vi "Zaber A Series Streaming.vi"() -> ()   [LabVIEW 2015]
doc: "Streaming lets you queue a number of commands to be completed in series. With multi-axis controllers the movement is co-ordinated to make lines, arcs, or circles. \n\nThis example allows interactive execution of some of the streaming commands. Some of the features will function with single axis streams."
uses:
  Zaber A Series.lvlib
  <vilib>/Utility/file.llb/Read Delimited Spreadsheet (string).vi
  Public/Action-Status/Streaming/Stream Line (FW7).vi
  Public/Action-Status/Streaming/Stream Arc (FW7).vi
  Public/Action-Status/Streaming/Stream Circle (FW7).vi
panel:
  in  "Quit":bool
  in  "End Stream":bool
  in  "Start Stream":bool
  in  "Stop":bool
  in  "Device Number":string
  in  "VISA resource name":refnum<visa-resource-name>
  in  "Home Axes":bool
  out "Port Open":bool
  out "Device supports streams":bool
  in  "Connect":bool
  in  "Close Port":bool
  out "Number of Stream Buffers Available":i32
  out "Number of Streams Available":i32
  in  "Stream Number":u8=1
  in  "Axis Numbers":u8[](array[numeric])=[1, 2]
  in  "Tab Control":enum32{"Stream Commands", "Command List"}(tab)
  in  "Position Units (0: microsteps)":u16(ring) items=["microsteps", "microns", "millimeters", "inches", "degrees"]
  in  "Microstep Size (0)":dbl
  in  "Line Endpoint":i64[](array[numeric])
  in  "Position Mode":u16(ring) items=["Absolute", "Relative"]
  in  "Line":bool
  in  "Circle":bool
  in  "Arc":bool
  in  "Direction":u16(ring) items=["Clockwise", "Counter-Clockwise"]
  in  "Center":i64[](array[numeric])
  in  "Arc End Point":i64[](array[numeric])
  in  "Send Stream List":bool
  in  "Import CSV":bool
  in  "Stream Commands":string[][](table)=[["stream 1 line rel 20000 20000"], ["stream 1 circle rel cw 10000 0"], ["stream 1 wait 2000"], ["stream 1 line abs 0 0"]]
  in  "file path (dialog if empty)":path
  # "(c) 2017 Zaber Technologies.  ALL RIGHTS RESERVED."
  # "This example demonstrates use of live streaming commands. \n\nFirst Open the port and Home all Axes. The VI will confirm if streams are supported on the device.\n\nNext, enter the Device Number, Stream Number (typically 1), and Axis Numbers (if only 1 axis, then right click on the second axis and select 'delete'). Press Start Stream to begin sending movements.\n\nThe Stream Commands tab allows you to send Lines, Arcs, and Circles. The Command List tab allows you to enter a series of stream commands, or load a list of them from a CSV, and run them in sequence."
  # "Movement"
  # "Lines"
  # "Arcs and Circles"
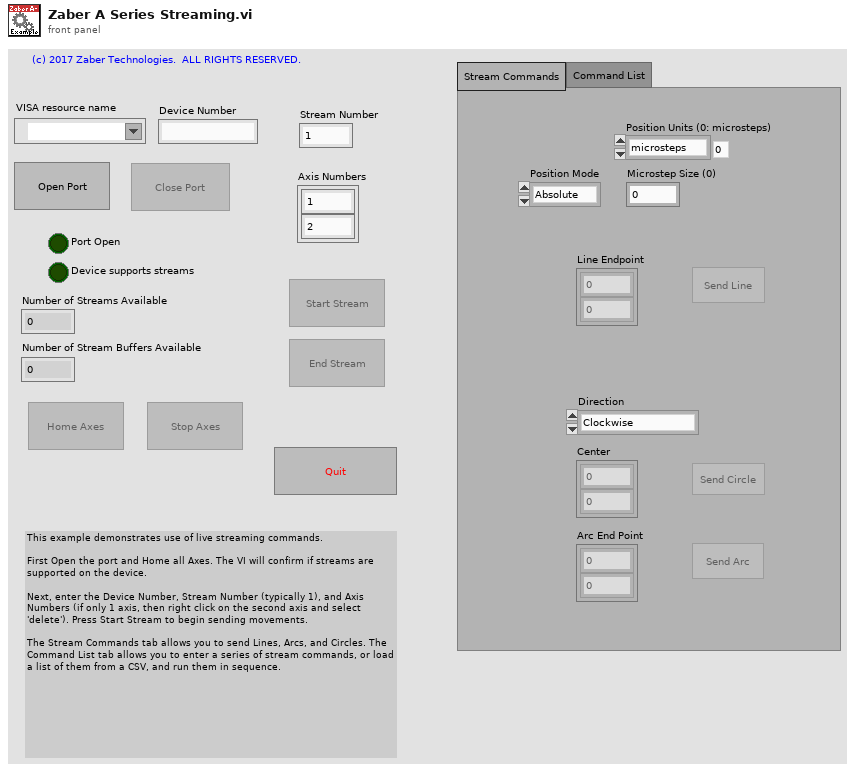
[diagram p1: front panel]
types:
  T1 = enum8{"Enabled", "Disabled", "Disabled and Grayed Out"}
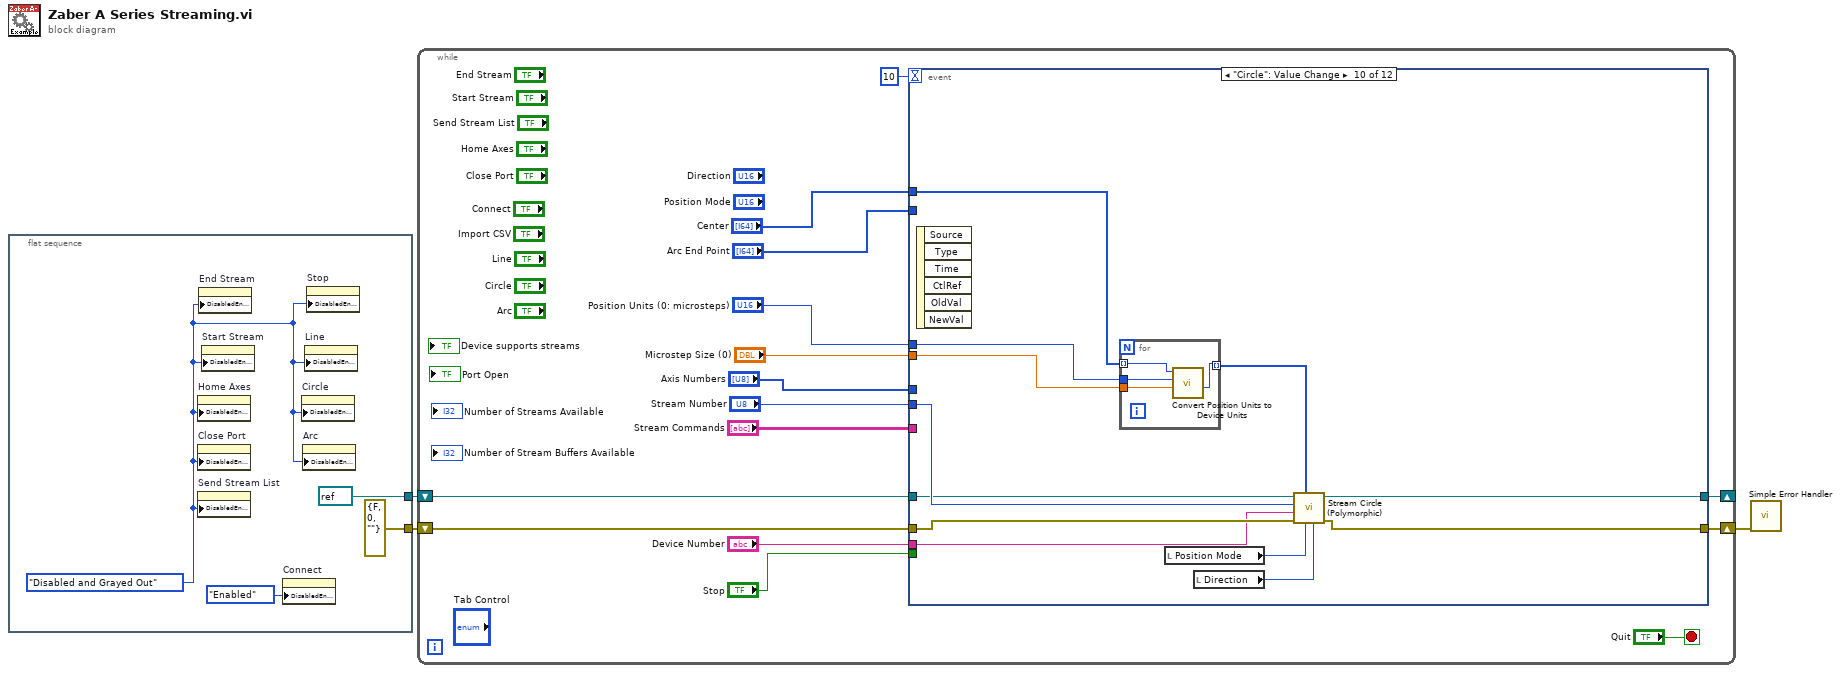
[diagram p0: block diagram]
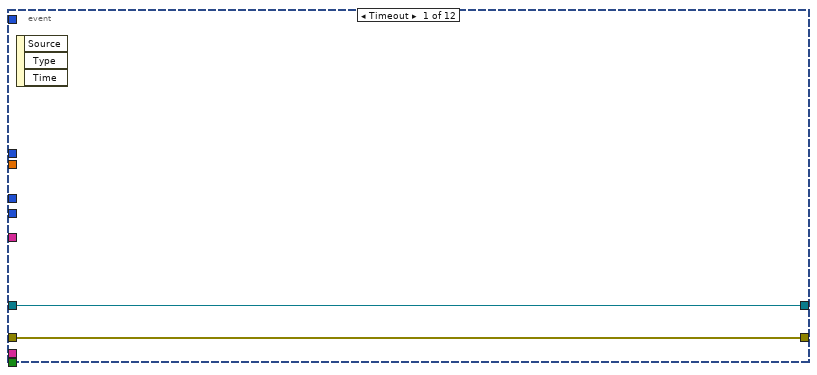
[diagram p2: hidden frame]
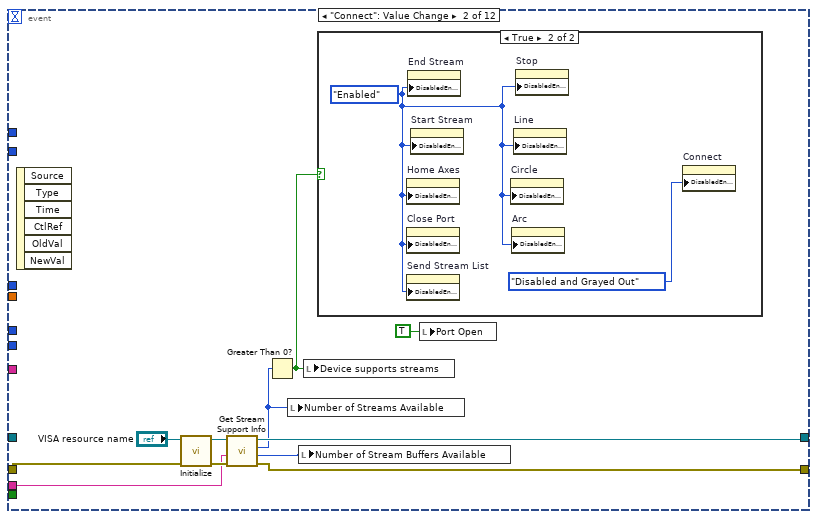
[diagram p3: hidden frame]
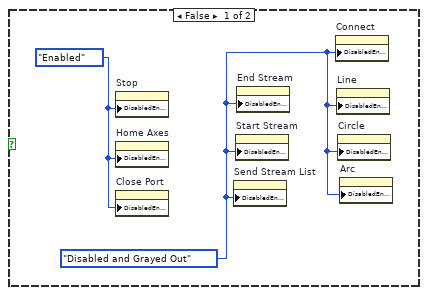
[diagram p4: hidden frame]
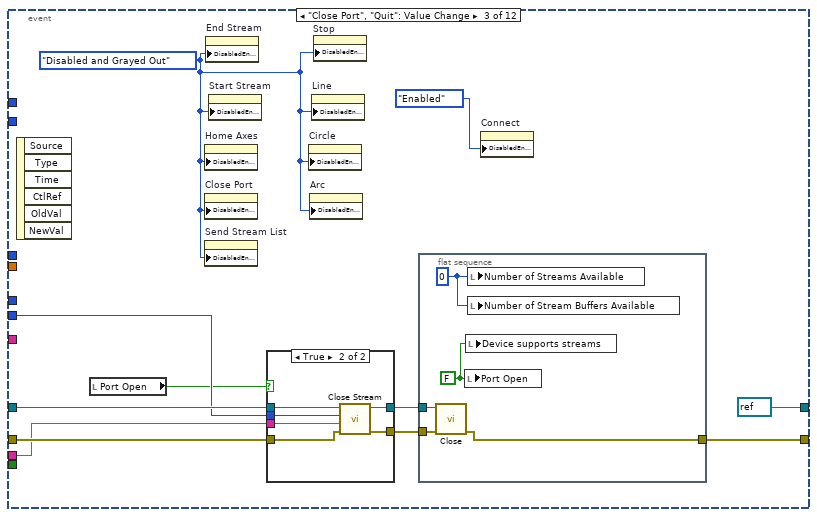
[diagram p5: hidden frame]
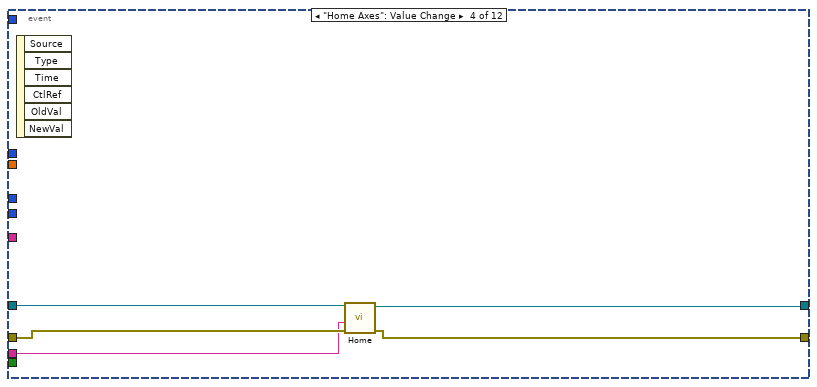
[diagram p7: hidden frame]
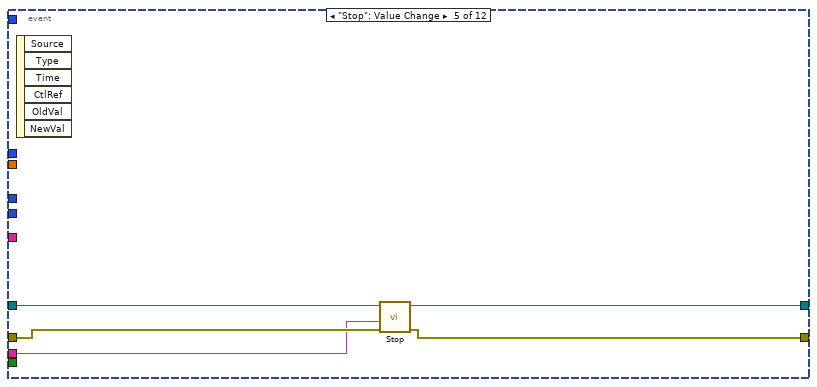
[diagram p8: hidden frame]
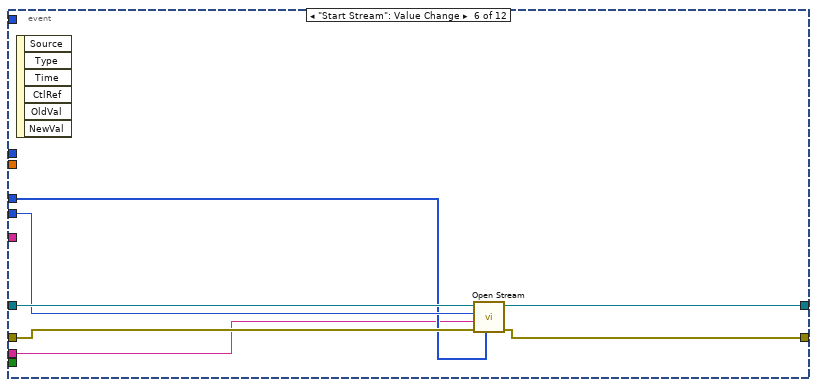
[diagram p9: hidden frame]
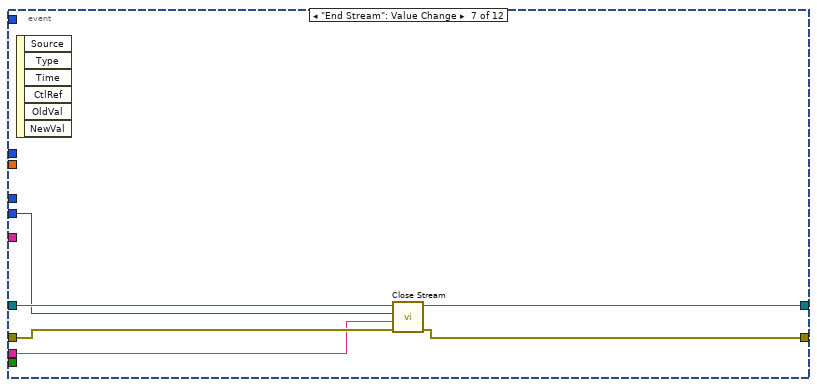
[diagram p10: hidden frame]
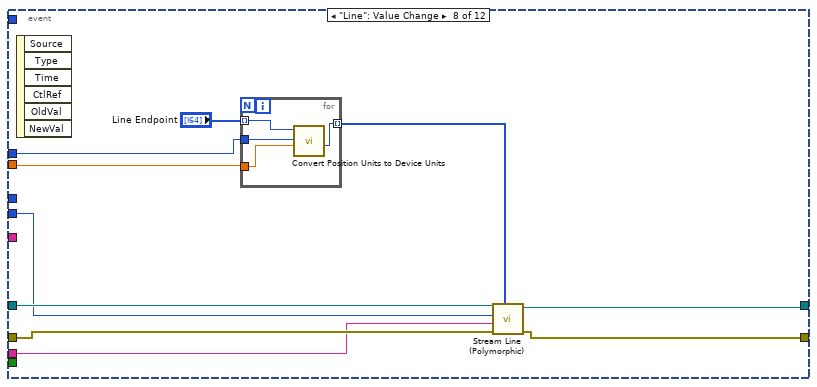
[diagram p11: hidden frame]
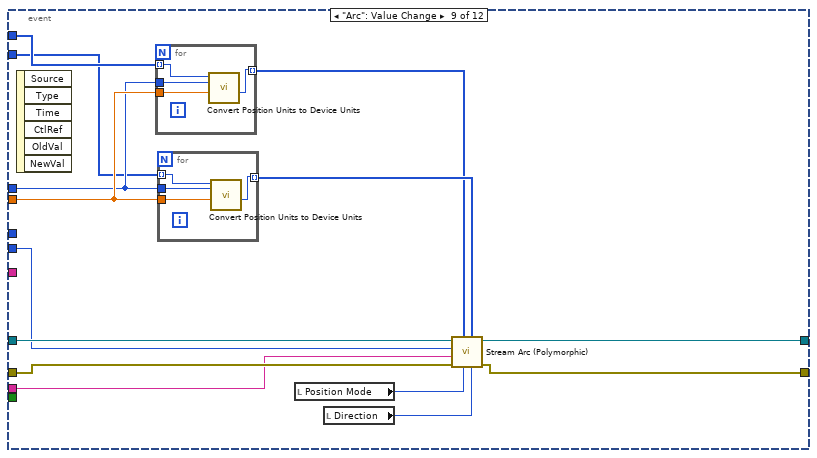
[diagram p12: hidden frame]
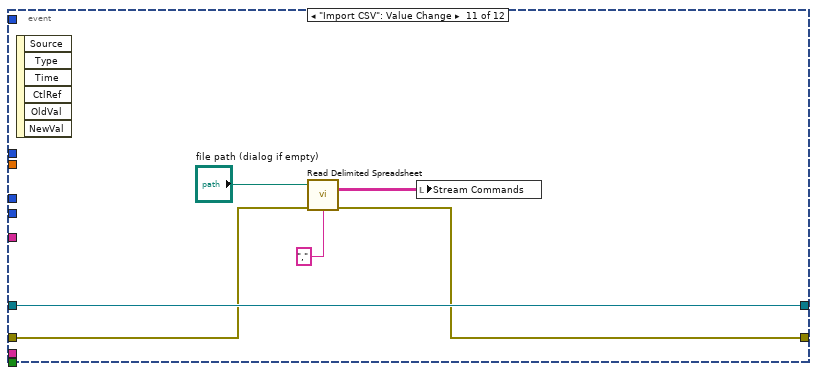
[diagram p13: hidden frame]
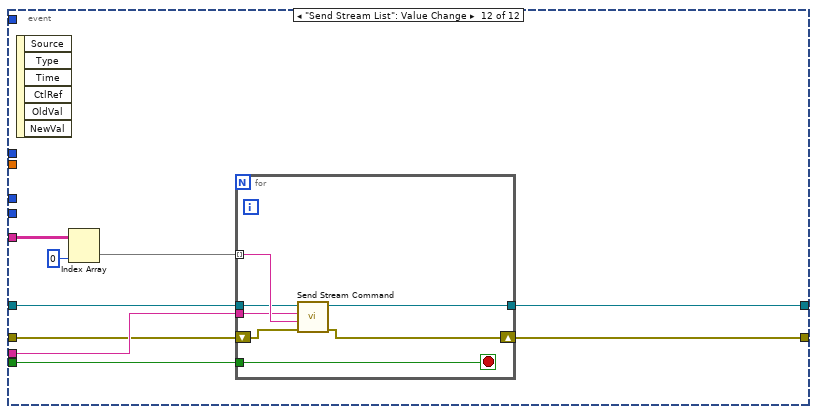
[diagram p14: hidden frame]
diagram:
  n1 = flat-sequence {
    tunnel: [errorcluster {"status"=FALSE, "code"=0, "source"=""} ("error out")] -> w3
    tunnel: [refnum<visa-resource-name> refnum ("VISA resource name out")] -> w2
    frame #0 {
      w5 = T1."Disabled and Grayed Out" ("Disabled")
      n2 = property on="Home Axes" class="Bool"("DisabledEnum"=w5) -> ()  [unwired: 2 in, 2 out]
      n3 = property on="Close Port" class="Bool"("DisabledEnum"=w5) -> ()  [unwired: 2 in, 2 out]
      n4 = property on="Send Stream List" class="Bool"("DisabledEnum"=w5) -> ()  [unwired: 2 in, 2 out]
      n5 = property on="End Stream" class="Bool"("DisabledEnum"=w5) -> ()  [unwired: 2 in, 2 out]
      n6 = property on="Start Stream" class="Bool"("DisabledEnum"=w5) -> ()  [unwired: 2 in, 2 out]
      n7 = property on="Connect" class="Bool"("DisabledEnum"=T1."Enabled" ("Disabled")) -> ()  [unwired: 2 in, 2 out]
      n8 = property on="Circle" class="Bool"("DisabledEnum"=w5) -> ()  [unwired: 2 in, 2 out]
      n9 = property on="Arc" class="Bool"("DisabledEnum"=w5) -> ()  [unwired: 2 in, 2 out]
      n10 = property on="Line" class="Bool"("DisabledEnum"=w5) -> ()  [unwired: 2 in, 2 out]
      n11 = property on="Stop" class="Bool"("DisabledEnum"=w5) -> ()  [unwired: 2 in, 2 out]
    }
  }
  n12 = while {
    shift-right: [w18] -> _
    shift-left: w2 -> [w17]
    shift-right: [w16] -> w1
    shift-left: w3 -> [w15]
    stop <- "Quit" stop-if-true
    n13 = event shown="[9] \"Circle\": Value Change" {
      selector: _ -> [_ _ _ _ _ _ _ _ _ _ _ _]
      dyn-events: _ -> [_ _ _ _ _ _ _ _ _ _ _ _]
      timeout: 10 -> [_ _ _ _ _ _ _ _ _ _ _ _]
      tunnel: "Stream Commands" -> [_ _ _ _ _ _ _ _ _ _ _ w153]
      tunnel: "Device Number" -> [_ w30 w44 w64 w69 w74 w81 w90 w105 w129 _ w150]
      tunnel: "Stop" -> [_ _ _ _ _ _ _ _ _ _ _ w149]
      tunnel: [w24 w31 refnum<visa-resource-name> refnum ("VISA resource name out") w67 w72 w80 w85 w93 w111 w130 w141 w148] -> w18
      tunnel: w17 -> [w24 _ w48 w68 w73 w79 w86 w94 w112 w133 w141 w147]
      tunnel: [w23 w32 w50 w65 w70 w77 w83 w91 w109 w131 w139 w146] -> w16
      tunnel: w15 -> [w23 w34 w46 w66 w71 w78 w84 w92 w110 w132 w140 w145]
      tunnel: "Stream Number" -> [_ _ w41 _ _ w76 w82 w89 w108 w134 _ _]
      tunnel: "Axis Numbers" -> [_ _ _ _ _ w75 _ _ _ _ _ _]
      tunnel: "Microstep Size (0)" -> [_ _ _ _ _ _ _ w88 w104 w125 _ _]
      tunnel: "Position Units (0: microsteps)" -> [_ _ _ _ _ _ _ w87 w103 w124 _ _]
      tunnel: "Center" -> [_ _ _ _ _ _ _ _ w102 w123 _ _]
      tunnel: "Arc End Point" -> [_ _ _ _ _ _ _ _ w101 _ _ _]
      event Timeout {
        n14 = event-data() -> ()  [unwired: 1 in, 3 out]
      }
      event "Connect": Value Change {
        n15 = event-data() -> ()  [unwired: 1 in, 6 out]
        n16 = call "Initialize.vi"("error in (no error)"=w34, "VISA resource name"="VISA resource name") -> ("error out"=w33:errorcluster, "VISA resource name out"=w35:refnum<visa-resource-name>)  [unwired: 8 in]
        n17 = call "Get Stream Support Info.vi"("error in (no error)"=w33, "Device Number"=w30, "VISA resource name"=w35) -> ("error out"=w32:errorcluster, "Number of Buffers"=w26:i32, "Number of Streams"=w25:i32, "VISA resource name out"=w31:refnum<visa-resource-name>)  [unwired: 5 in]
        n18 = Greater Than 0?(x=w25) -> (x > 0?=w27:bool)
        n19 = local write "Number of Streams Available"(w25) -> ()
        n20 = local write "Number of Stream Buffers Available"(w26) -> ()
        n21 = local write "Device supports streams"(w27) -> ()
        n22 = case shown="True" w27 {
          frame False {
            w36 = T1."Disabled and Grayed Out" ("Disabled")
            w37 = T1."Enabled" ("Disabled")
            n23 = property on="Stop" class="Bool"("DisabledEnum"=w37) -> ()  [unwired: 2 in, 2 out]
            n24 = property on="Home Axes" class="Bool"("DisabledEnum"=w37) -> ()  [unwired: 2 in, 2 out]
            n25 = property on="Close Port" class="Bool"("DisabledEnum"=w37) -> ()  [unwired: 2 in, 2 out]
            n26 = property on="Send Stream List" class="Bool"("DisabledEnum"=w36) -> ()  [unwired: 2 in, 2 out]
            n27 = property on="Start Stream" class="Bool"("DisabledEnum"=w36) -> ()  [unwired: 2 in, 2 out]
            n28 = property on="End Stream" class="Bool"("DisabledEnum"=w36) -> ()  [unwired: 2 in, 2 out]
            n29 = property on="Connect" class="Bool"("DisabledEnum"=w36) -> ()  [unwired: 2 in, 2 out]
            n30 = property on="Line" class="Bool"("DisabledEnum"=w36) -> ()  [unwired: 2 in, 2 out]
            n31 = property on="Circle" class="Bool"("DisabledEnum"=w36) -> ()  [unwired: 2 in, 2 out]
            n32 = property on="Arc" class="Bool"("DisabledEnum"=w36) -> ()  [unwired: 2 in, 2 out]
          }
          frame True {
            w39 = T1."Enabled" ("Disabled")
            n33 = property on="Home Axes" class="Bool"("DisabledEnum"=w39) -> ()  [unwired: 2 in, 2 out]
            n34 = property on="Close Port" class="Bool"("DisabledEnum"=w39) -> ()  [unwired: 2 in, 2 out]
            n35 = property on="Send Stream List" class="Bool"("DisabledEnum"=w39) -> ()  [unwired: 2 in, 2 out]
            n36 = property on="End Stream" class="Bool"("DisabledEnum"=w39) -> ()  [unwired: 2 in, 2 out]
            n37 = property on="Start Stream" class="Bool"("DisabledEnum"=w39) -> ()  [unwired: 2 in, 2 out]
            n38 = property on="Circle" class="Bool"("DisabledEnum"=w39) -> ()  [unwired: 2 in, 2 out]
            n39 = property on="Arc" class="Bool"("DisabledEnum"=w39) -> ()  [unwired: 2 in, 2 out]
            n40 = property on="Line" class="Bool"("DisabledEnum"=w39) -> ()  [unwired: 2 in, 2 out]
            n41 = property on="Stop" class="Bool"("DisabledEnum"=w39) -> ()  [unwired: 2 in, 2 out]
            n42 = property on="Connect" class="Bool"("DisabledEnum"=T1."Disabled and Grayed Out" ("Disabled")) -> ()  [unwired: 2 in, 2 out]
          }
        }
        n43 = local write "Port Open"(TRUE ("Port Open")) -> ()
      }
      event "Close Port", "Quit": Value Change {
        w43 = T1."Disabled and Grayed Out" ("Disabled")
        n44 = event-data() -> ()  [unwired: 1 in, 6 out]
        n45 = local read "Port Open"() -> (w40:bool)
        n46 = property on="Home Axes" class="Bool"("DisabledEnum"=w43) -> ()  [unwired: 2 in, 2 out]
        n47 = property on="Close Port" class="Bool"("DisabledEnum"=w43) -> ()  [unwired: 2 in, 2 out]
        n48 = property on="Send Stream List" class="Bool"("DisabledEnum"=w43) -> ()  [unwired: 2 in, 2 out]
        n49 = property on="End Stream" class="Bool"("DisabledEnum"=w43) -> ()  [unwired: 2 in, 2 out]
        n50 = property on="Start Stream" class="Bool"("DisabledEnum"=w43) -> ()  [unwired: 2 in, 2 out]
        n51 = case shown="True" w40 {
          tunnel: w48 -> [w57 w63]
          tunnel: [w57 w62] -> w47
          tunnel: w46 -> [w56 w61]
          tunnel: [w56 w60] -> w45
          tunnel: w44 -> [_ w59]
          tunnel: w41 -> [_ w58]
          frame False {
          }
          frame True {
            n52 = call "Close Stream.vi"("error in (no error)"=w61, "Device Number"=w59, "Stream Number (1)"=w58, "VISA resource name"=w63) -> ("error out"=w60:errorcluster, "VISA resource name out"=w62:refnum<visa-resource-name>)  [unwired: 6 in]
          }
        }
        n53 = property on="Circle" class="Bool"("DisabledEnum"=w43) -> ()  [unwired: 2 in, 2 out]
        n54 = property on="Arc" class="Bool"("DisabledEnum"=w43) -> ()  [unwired: 2 in, 2 out]
        n55 = property on="Line" class="Bool"("DisabledEnum"=w43) -> ()  [unwired: 2 in, 2 out]
        n56 = property on="Stop" class="Bool"("DisabledEnum"=w43) -> ()  [unwired: 2 in, 2 out]
        n57 = flat-sequence {
          tunnel: [w55] -> w50
          tunnel: w47 -> [w54]
          tunnel: w45 -> [w53]
          frame #0 {
            w51 = 0 ("Number of Streams Available")
            w52 = FALSE ("Port Open")
            n58 = call "Close.vi"("error in (no error)"=w53, "VISA resource name"=w54) -> ("error out"=w55:errorcluster)  [unwired: 9 in]
            n59 = local write "Port Open"(w52) -> ()
            n60 = local write "Device supports streams"(w52) -> ()
            n61 = local write "Number of Streams Available"(w51) -> ()
            n62 = local write "Number of Stream Buffers Available"(w51) -> ()
          }
        }
        n63 = property on="Connect" class="Bool"("DisabledEnum"=T1."Enabled" ("Disabled")) -> ()  [unwired: 2 in, 2 out]
      }
      event "Home Axes": Value Change {
        n64 = event-data() -> ()  [unwired: 1 in, 6 out]
        n65 = call "Home.vi"("error in (no error)"=w66, "Device and Axis"=w64, "VISA resource name"=w68) -> ("error out"=w65:errorcluster, "VISA resource name out"=w67:refnum<visa-resource-name>)  [unwired: 7 in]
      }
      event "Stop": Value Change {
        n66 = event-data() -> ()  [unwired: 1 in, 6 out]
        n67 = call "Stop.vi"("error in (no error)"=w71, "Device and Axis"=w69, "VISA resource name"=w73) -> ("error out"=w70:errorcluster, "VISA resource name out"=w72:refnum<visa-resource-name>)  [unwired: 7 in]
      }
      event "Start Stream": Value Change {
        n68 = event-data() -> ()  [unwired: 1 in, 6 out]
        n69 = call "Open Stream.vi"("Axis Numbers (1,2)"=w75, "error in (no error)"=w78, "Device Number"=w74, "Stream Number (1)"=w76, "VISA resource name"=w79) -> ("error out"=w77:errorcluster, "VISA resource name out"=w80:refnum<visa-resource-name>)  [unwired: 5 in]
      }
      event "End Stream": Value Change {
        n70 = event-data() -> ()  [unwired: 1 in, 6 out]
        n71 = call "Close Stream.vi"("error in (no error)"=w84, "Device Number"=w81, "Stream Number (1)"=w82, "VISA resource name"=w86) -> ("error out"=w83:errorcluster, "VISA resource name out"=w85:refnum<visa-resource-name>)  [unwired: 6 in]
      }
      event "Line": Value Change {
        n72 = event-data() -> ()  [unwired: 1 in, 6 out]
        n73 = for {
          tunnel: "Line Endpoint" -> [w100] mode=indexing
          tunnel: [w97] -> w96 mode=indexing
          tunnel: w88 -> [w99]
          tunnel: w87 -> [w98]
          n74 = call "Convert Position Units to Device Units.vi"("Microstep Size (0)"=w99, "Units (0: microsteps)"=w98, "Position (0)"=w100) -> ("Device Position (64-bit)"=w97:i64)  [unwired: 6 in, 2 out]
        }
        n75 = call-poly "Stream Line (Polymorphic).vi"("Coordinates"=w96, "error in (no error)"=w92, "Device Number"=w90, "Stream Number (1)"=w89, "VISA resource name"=w94) -> ("error out"=w91:errorcluster, "VISA resource name out"=w93:refnum<visa-resource-name>)  [unwired: 5 in]
      }
      event "Arc": Value Change {
        n76 = event-data() -> ()  [unwired: 1 in, 6 out]
        n77 = for {
          tunnel: [w119] -> w113 mode=indexing
          tunnel: w104 -> [w122]
          tunnel: w103 -> [w121]
          tunnel: w102 -> [w120] mode=indexing
          n78 = call "Convert Position Units to Device Units.vi"("Microstep Size (0)"=w122, "Units (0: microsteps)"=w121, "Position (0)"=w120) -> ("Device Position (64-bit)"=w119:i64)  [unwired: 6 in, 2 out]
        }
        n79 = for {
          tunnel: [w115] -> w114 mode=indexing
          tunnel: w104 -> [w118]
          tunnel: w103 -> [w117]
          tunnel: w101 -> [w116] mode=indexing
          n80 = call "Convert Position Units to Device Units.vi"("Microstep Size (0)"=w118, "Units (0: microsteps)"=w117, "Position (0)"=w116) -> ("Device Position (64-bit)"=w115:i64)  [unwired: 6 in, 2 out]
        }
        n81 = local read "Position Mode"() -> (w107:u16)
        n82 = local read "Direction"() -> (w106:u16)
        n83 = call-poly "Stream Arc (Polymorphic).vi"("Direction (0: clockwise)"=w106, "End Point"=w114, "Position Mode (0: absolute)"=w107, "Center Point"=w113, "error in (no error)"=w110, "Device Number"=w105, "Stream Number (1)"=w108, "VISA resource name"=w112) -> ("error out"=w109:errorcluster, "VISA resource name out"=w111:refnum<visa-resource-name>)  [unwired: 2 in]
      }
      event "Circle": Value Change {
        n84 = event-data() -> ()  [unwired: 1 in, 6 out]
        n85 = for {
          tunnel: [w135] -> w128 mode=indexing
          tunnel: w125 -> [w138]
          tunnel: w124 -> [w137]
          tunnel: w123 -> [w136] mode=indexing
          n86 = call "Convert Position Units to Device Units.vi"("Microstep Size (0)"=w138, "Units (0: microsteps)"=w137, "Position (0)"=w136) -> ("Device Position (64-bit)"=w135:i64)  [unwired: 6 in, 2 out]
        }
        n87 = local read "Position Mode"() -> (w127:u16)
        n88 = local read "Direction"() -> (w126:u16)
        n89 = call-poly "Stream Circle (Polymorphic).vi"("Direction (0: clockwise)"=w126, "Position Mode (0: absolute)"=w127, "Center"=w128, "error in (no error)"=w132, "Device Number"=w129, "Stream Number (1)"=w134, "VISA resource name"=w133) -> ("error out"=w131:errorcluster, "VISA resource name out"=w130:refnum<visa-resource-name>)  [unwired: 3 in]
      }
      event "Import CSV": Value Change {
        n90 = event-data() -> ()  [unwired: 1 in, 6 out]
        n91 = call-poly <vilib>:"Read Delimited Spreadsheet.vi"("file path (dialog if empty)"="file path (dialog if empty)", "error in (no error)"=w140, "delimiter (\\t)"="," ("delimiter (\\t)")) -> ("all rows"=w144:string[][], "error out"=w139:errorcluster)  [unwired: 7 in, 4 out]
        n92 = local write "Stream Commands"(w144) -> ()
      }
      event "Send Stream List": Value Change {
        n93 = event-data() -> ()  [unwired: 1 in, 6 out]
        n94 = Index Array(array=w153, index (col)=0 ("disabled index (col)")) -> (element=w151:string[])  [unwired: 1 in]
        n95 = for {
          tunnel: w151 -> [w160] mode=indexing
          tunnel: w150 -> [w159]
          tunnel: w149 -> [w158]
          tunnel: [w157] -> w148
          tunnel: w147 -> [w156]
          shift-right: [w155] -> w146
          shift-left: w145 -> [w154]
          stop <- w158 stop-if-true
          n96 = call "Send Stream Command.vi"("error in (no error)"=w154, "Command"=w160, "Device Number"=w159, "VISA resource name"=w156) -> ("error out"=w155:errorcluster, "VISA resource name out"=w157:refnum<visa-resource-name>)  [unwired: 6 in]
        }
      }
    }
  }
  n97 = call <vilib>:"Simple Error Handler.vi"("error in (no error)"=w1) -> ()  [unwired: 4 in, 5 out]
